vi "Complex To Cartesian - RM.vi"(0 "Real Matrix R + 0i":T1) -> (1 "Real Matrix R":T1, 2 "Real Matrix I (0)":T1)   [LabVIEW 2024, in "NI_Matrix.lvlib"]
doc: "Breaks a complex number into its rectangular components."
uses:
  NI_Matrix.lvlib
  RealMatrix.ctl
  Array To Matrix - RA2.vi
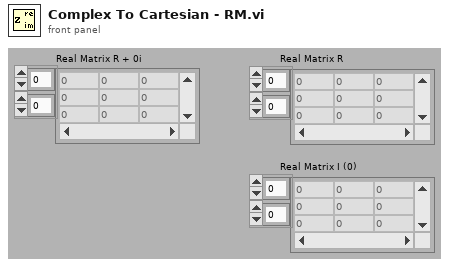
[diagram p1: front panel]
types:
  T1 = typedef "NI_Matrix.lvlib/RealMatrix.ctl" = dbl[][]
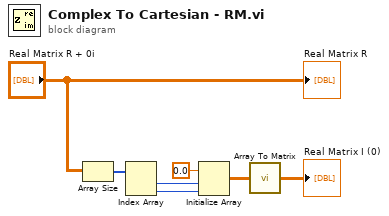
[diagram p0: block diagram]
diagram:
  n1 = Array Size(array="Real Matrix R + 0i") -> (size(s)=w6:i32[])
  n2 = Index Array(array=w6) -> (element #1=w4:i32, element #2=w3:i32)  [unwired: 2 in]
  n3 = Initialize Array(0.0 ("element"), w4, w3) -> (w2:dbl[][])
  n4 = call-poly "Array To Matrix.vi"("Real 2D Array"=w2) -> ("Real Matrix"=→"Real Matrix I (0)":T1)
  "Real Matrix R" <- "Real Matrix R + 0i"
